vi "Set function and range.vi"(8 "error in":errorcluster, 9 "Range number (0)":u16 max=9, 10 "Function (F0 - V DC)":T1(ring), 11 "VISA resource name":refnum<visa-resource-name>) -> (0 "error out":errorcluster, 3 "VISA resource name out":refnum<visa-resource-name>)   [LabVIEW 2013, in "Datron D4xxx.lvlib"]
doc: "Sets function and reange at once."
uses:
  Datron D4xxx.lvlib
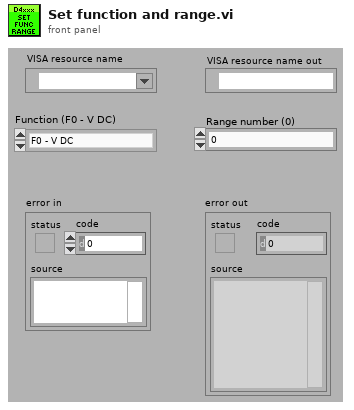
[diagram p1: front panel]
types:
  T1 = enum16{"F0 - V DC", "F1 - V AC", "F2 - A DC", "F3 - A AC", "F4 - R", "F5 - V WB"}
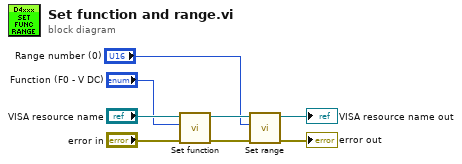
[diagram p0: block diagram]
diagram:
  n1 = call "Set function.vi"("error in"="error in", "Function (F0 - V DC)"="Function (F0 - V DC)", "VISA resource name"="VISA resource name") -> ("error out"=w5:errorcluster, "VISA resource name out"=w6:refnum<visa-resource-name>)  [unwired: 7 in]
  n2 = call "Set range.vi"("error in"=w5, "Range number {0 to 9}"="Range number (0)", "VISA resource name"=w6) -> ("error out"=→"error out":errorcluster, "VISA resource name out"=→"VISA resource name out":refnum<visa-resource-name>)  [unwired: 7 in]
